vi "initialize comm references.vi"(8 "error in (no error)":errorcluster, 11 "sequencer name":string) -> (0 "error out":errorcluster, 1 "message queue out":T1, 2 "cmd queue out":T1, 3 "config notifier out":refnum<notifier>)   [LabVIEW 2015, in "Simple Sequencer TBM runtime.lvclass"]
doc: "Initializes the communication queues and notifiers, useing the sequencer name, in order to communicate with the sequencer's programmatic API."
uses:
  Simple Sequencer TBM runtime.lvclass
  <vilib>/NI/AMC/Message Queue.ctl
  <vilib>/NI/AMC/Message.ctl
  <vilib>/NI/Tools/Keyed Array/KeyedArray.ctl
  configuration/Simple Sequencer TBM configuration.lvclass
  <vilib>/NI/AMC/AMC.lvlib
  <vilib>/NI/Tools/Keyed Array/Tools_KeyedArray.lvlib
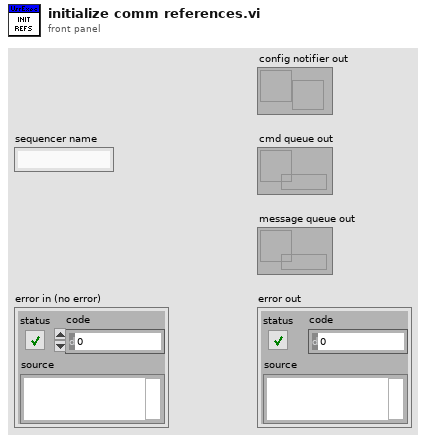
[diagram p1: front panel]
types:
  T1 = typedef "AMC.lvlib/Message Queue.ctl" = refnum<queue>
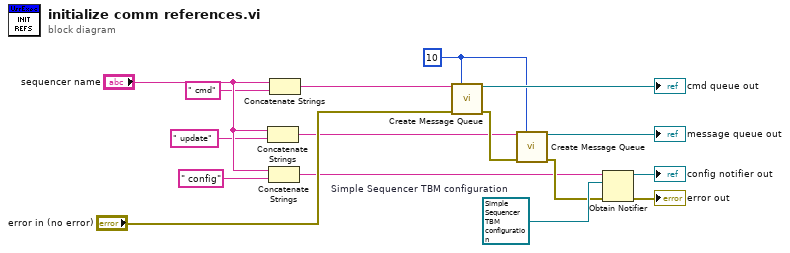
[diagram p0: block diagram]
diagram:
  w1 = 10 ("max queue size (-1, unlimited)")
  w13 = refnum<class "Simple Sequencer TBM configuration.lvclass"> refnum  # Simple Sequencer TBM configuration
  n1 = Concatenate Strings("sequencer name", " update" ("string")) -> (w7:string)
  n2 = Concatenate Strings("sequencer name", " config" ("string")) -> (w8:string)
  n3 = Concatenate Strings("sequencer name", " cmd" ("string")) -> (w6:string)
  n4 = call <vilib>:"Create Message Queue.vi"("message queue name"=w6, "max queue size (-1, unlimited)"=w1, "error in"="error in (no error)") -> ("message queue out"=→"cmd queue out":T1, "error out"=w9:errorcluster)  [unwired: 11 in]
  n5 = call <vilib>:"Create Message Queue.vi"("message queue name"=w7, "max queue size (-1, unlimited)"=w1, "error in"=w9) -> ("message queue out"=→"message queue out":T1, "error out"=w10:errorcluster)  [unwired: 11 in]
  n6 = Obtain Notifier(name (unnamed)=w8, notification data type=w13, error in (no error)=w10) -> (notifier out=→"config notifier out":refnum<notifier>, error out=→"error out":errorcluster)  [unwired: 1 in, 1 out]
